vi "Pockels-Set modulation exit level.vi"(9 "Pockels control value (V)":dbl, 11 "task/channels in":refnum<k21>) -> (0 "error out":errorcluster, 3 "task out":refnum<k21>)   [LabVIEW 2020]
uses:
  Typedefs/Functional Global Default States.ctl
  <vilib>/DAQmx/write.llb/DAQmx Write (Analog 1D DBL 1Chan NSamp).vi
  Globals/gl_Pockels control globals.vi
  <vilib>/DAQmx/miscellaneous.llb/DAQmx Fill In Error Info.vi
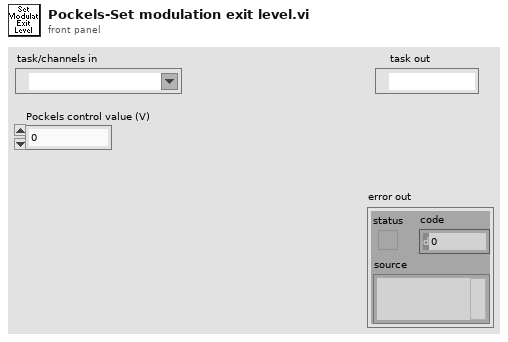
[diagram p1: front panel]
types:
  T1 = typedef "Functional Global Default States.ctl" = enum16{"Read", "Write", "Clear"}
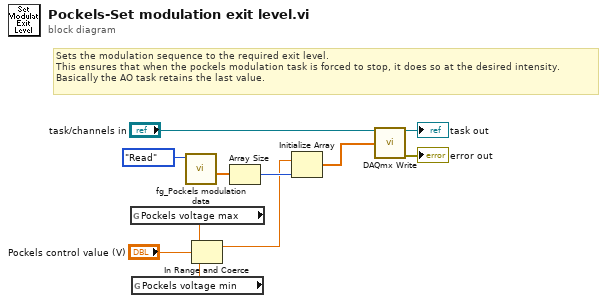
[diagram p0: block diagram]
diagram:
  # "Sets the modulation sequence to the required exit level.\nThis ensures that when the pockels modulation task is forced to stop, it does so at the desired intensity.\nBasically the AO task retains the last value."
  n1 = global read "gl_Pockels control globals.vi" "Pockels voltage max"() -> (w9:dbl)
  n2 = global read "gl_Pockels control globals.vi" "Pockels voltage min"() -> (w8:dbl)
  n3 = call "fg_Pockels modulation data.vi"("Function"=Functional_Global_Default_States."Read") -> ("Pockels modulation data out"=w6:dbl[])  [unwired: 10 in]
  n4 = In Range and Coerce(upper limit=w9, x="Pockels control value (V)", lower limit=w8) -> (coerced(x)=w4:dbl)  [unwired: 1 out]
  n5 = Array Size(array=w6) -> (size(s)=w5:i32)
  n6 = Initialize Array(w4, w5) -> (w3:dbl[])
  n7 = call-poly <vilib>:"DAQmx Write.vi"("task/channels in"="task/channels in", "data"=w3) -> ("task out"=→"task out":refnum<k21>, "error out"=→"error out":errorcluster)  [unwired: 11 in, 1 out]
